vi "周期设置.vi"(11 "定时控制参数输入":T1) -> (3 "定时控制参数输出":T1)   [LabVIEW 2016, in "CODCr库.lvlib"]
panel:
  out "选项卡控件":enum32{"定点启动", "间隔启动"}(tab)
  in  "24H周期设置":bool[](xcontrol)
  in  "定时间隔":dbl
  in  "确定":bool
  in  "取消":bool
  in  "定时功能启用":bool
  in  "周期设置类型":enum16{"定点启动", "间隔启动"}(ring)
  in  "仪器测试类型":enum16{"水样测试", "标样核查", "空白测试", "跨度核查"}(ring)
  # "仪器测试类型："
  # "周期设置类型："
  # "请输入定时启动间隔"
  # "min"
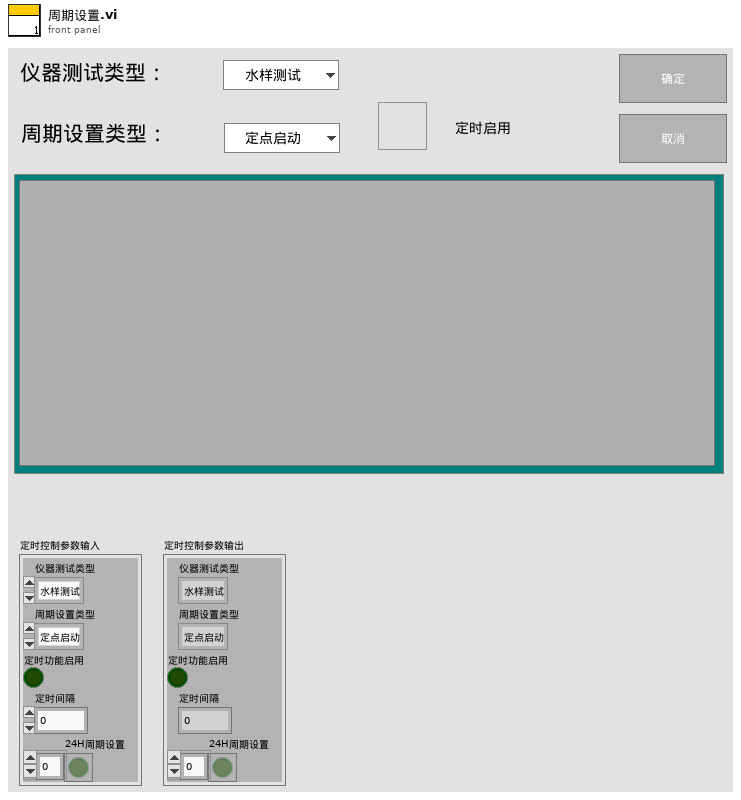
[diagram p1: front panel]
types:
  T1 = cluster{"仪器测试类型":enum16{"水样测试", "标样核查", "空白测试", "跨度核查"}, "周期设置类型":enum16{"定点启动", "间隔启动"}, "定时功能启用":bool, "定时间隔":dbl, "24H周期设置":bool[]}
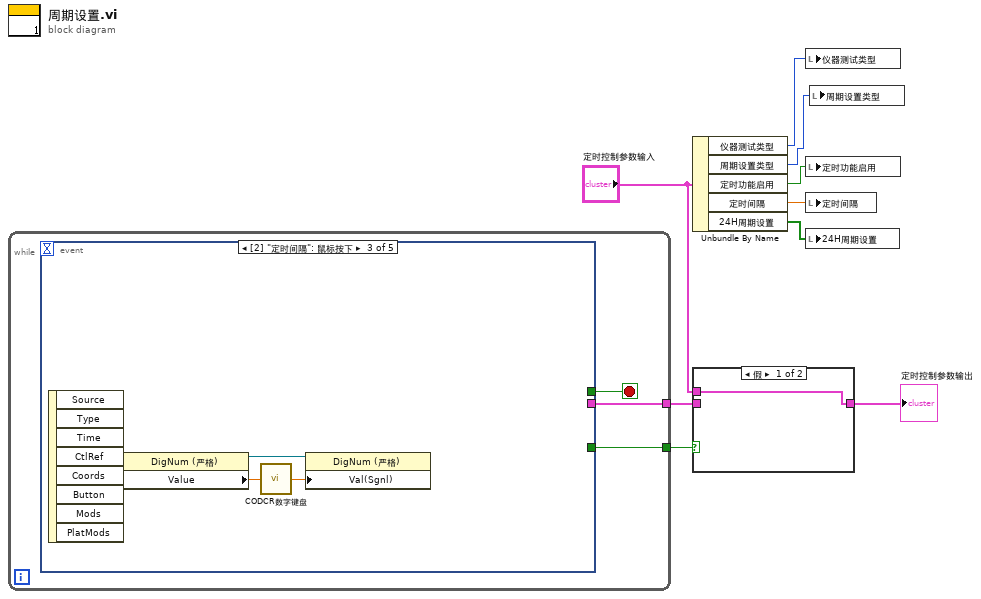
[diagram p0: block diagram]
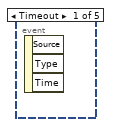
[diagram p3: hidden frame]
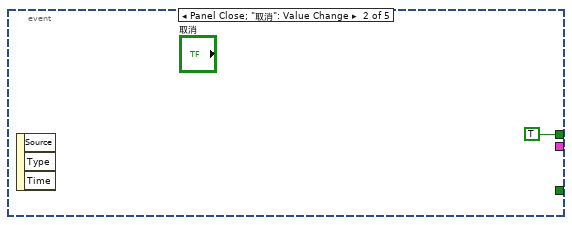
[diagram p4: hidden frame]
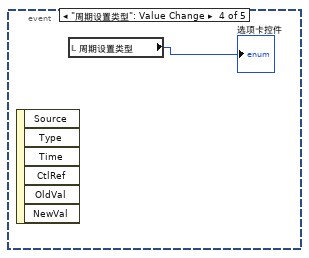
[diagram p5: hidden frame]
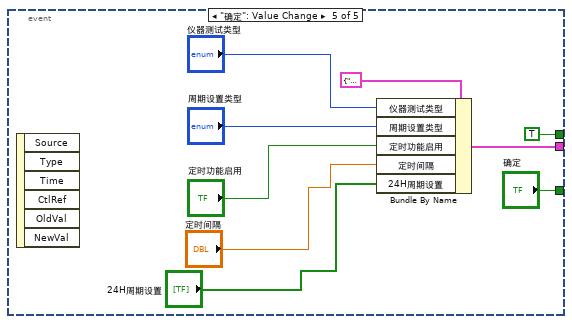
[diagram p6: hidden frame]
diagram:
  n1 = while {
    tunnel: [w11] -> w6
    tunnel: [w10] -> w7
    stop <- w12 stop-if-true
    n2 = event shown="[2] \"定时间隔\": 鼠标按下" {
      selector: _ -> [_ _ _ _ _]
      dyn-events: _ -> [_ _ _ _ _]
      timeout: _ -> [_ _ _ _ _]
      tunnel: [_ TRUE _ _ TRUE] -> w12
      tunnel: [_ _ _ _ w23] -> w11
      tunnel: [_ _ _ _ "确定"] -> w10
      event Timeout {
        n3 = event-data() -> ()  [unwired: 1 in, 3 out]
      }
      event Panel Close; "取消": Value Change {
        n4 = event-data() -> ()  [unwired: 1 in, 3 out]
      }
      event "定时间隔": Mouse Down {
        n5 = event-data() -> ("CtlRef"=w14:refnum<vi>)  [unwired: 1 in, 7 out]
        n6 = property class="DigNum (严格)"(reference=w14) -> (reference out=w15:refnum<vi>, "Value"=w17:dbl)  [unwired: 1 in, 1 out]
        n7 = call "CODCR数字键盘.vi"("OldNumber"=w17) -> ("NewNumber"=w16:sgl)
        n8 = property class="DigNum (严格)"(reference=w15, "Val(Sgnl)"=w16) -> ()  [unwired: 1 in, 2 out]
      }
      event "周期设置类型": Value Change {
        n9 = event-data() -> ()  [unwired: 1 in, 6 out]
        n10 = local read "周期设置类型"() -> (→"选项卡控件":enum16{"定点启动", "间隔启动"})
      }
      event "确定": Value Change {
        n11 = event-data() -> ()  [unwired: 1 in, 6 out]
        n12 = Bundle By Name(cluster=T1 {"仪器测试类型"=enum."水样测试", "周期设置类型"=enum."定点启动", "定时功能启用"=FALSE, "定时间隔"=0.0, "24H周期设置"=[]} ("定时控制"), "仪器测试类型"="仪器测试类型", "周期设置类型"="周期设置类型", "定时功能启用"="定时功能启用", "定时间隔"="定时间隔", "24H周期设置"="24H周期设置") -> (w23:T1)
      }
    }
  }
  n13 = Unbundle By Name("定时控制参数输入") -> ("仪器测试类型"=w9:enum16{"水样测试", "标样核查", "空白测试", "跨度核查"}, "周期设置类型"=w3:enum16{"定点启动", "间隔启动"}, "定时功能启用"=w8:bool, "定时间隔"=w2:dbl, "24H周期设置"=w1:bool[])
  n14 = case shown="假" w7 {
    tunnel: w6 -> [_ w29]
    tunnel: [w28 w29] -> w5
    tunnel: "定时控制参数输入" -> [w28 _]
    frame False {
    }
    frame True {
    }
  }
  "定时控制参数输出" <- w5
  n15 = local write "仪器测试类型"(w9) -> ()
  n16 = local write "定时功能启用"(w8) -> ()
  n17 = local write "定时间隔"(w2) -> ()
  n18 = local write "24H周期设置"(w1) -> ()
  n19 = local write "周期设置类型"(w3) -> ()
